vi "Actor Core.vi"(8 "error in":errorcluster, 11 "Form Model in":refnum<class "Form Model.lvclass">) -> (0 "error out":errorcluster, 3 "Actor out":refnum<class "Actor.lvclass">)   [LabVIEW 2020, in "Form Model.lvlib" / "Form Model.lvclass"]
doc: "(<B>Filename</B>: Actor Framework.lvlib:Actor.lvclass:Actor Core.vi)\n\nReceives messages to the actor, reacts to them, and initiates any error handling that may shut the actor down.\n\nDescendant classes may override this VI to append parallel tasks for the actor to complete while it handles messages. Overrides use the Call Parent Class Method node."
uses:
  Form Model.lvclass
  C:/Program Files (x86)/National Instruments/LabVIEW 2020/vi.lib/ActorFramework/Actor/Actor.lvclass
  <vilib>/ActorFramework/Actor/Actor.lvclass
  Form Model.lvclass/Form Model.ctl
  Forms Controller/Form Controller/Panel Form Controller.lvclass
  C:/Program Files (x86)/National Instruments/LabVIEW 2020/vi.lib/MGI/Panel Manager/Panel Actor/Panel Actor/Panel Actor.lvclass
  <vilib>/MGI/Panel Manager/Panel Actor/Panel Actor/Launch as Nested Actor.vi
  Form Model Configuration/Form Model Configuration Class/Form Model Configuration.lvclass
  Form Model Interfaces/Model Panel Logic Interface/Model Panel Logic.lvclass
  <vilib>/MGI/Monitored Actor/Monitored Actor/Monitored Actor/Monitored Actor.lvclass
  <vilib>/MGI/Panel Manager/Panel Actor/Panel Actor/Panel Actor.lvclass
  C:/Program Files (x86)/National Instruments/LabVIEW 2020/vi.lib/MGI/Monitored Actor/Monitored Actor/Monitored Actor/Monitored Actor.lvclass
  C:/Users/User/Desktop/Raman Program/Database OOP/source/Forms AF/Forms Controller/Form Controller/Panel Form Controller.lvclass
  C:/Users/User/Desktop/Raman Program/Database OOP/source/Forms AF/Forms Model/Form Model Actor/Form Model.lvclass
  C:/Users/User/Desktop/Raman Program/Database OOP/source/Forms AF/Forms Model/Form Model Interfaces/Form Model Messages/Form Model Messages.lvclass
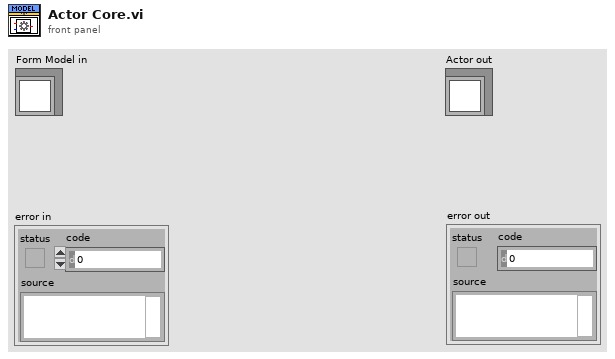
[diagram p1: front panel]
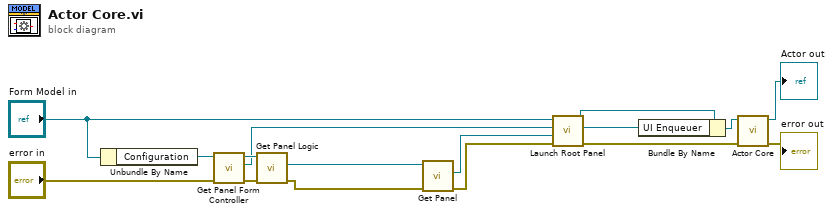
[diagram p0: block diagram]
diagram:
  n1 = Unbundle By Name("Form Model in") -> ("Configuration"=w7:refnum<class "Form Model Configuration.lvclass">)
  n2 = call-dynamic "Get Panel Form Controller.vi"("error in (no error)"="error in", "Form Model Configuration in"=w7) -> ("error out"=w5:errorcluster, "Panel Form Controller"=w8:refnum<class "Panel Form Controller.lvclass">, "Form Model Configuration out"=w9:refnum<class "Form Model Configuration.lvclass">)  [unwired: 7 in]
  n3 = call-dynamic "Get Panel Logic.vi"("error in (no error)"=w5, "Form Model Configuration in"=w9) -> ("error out"=w2:errorcluster, "Panel Logic"=w4:refnum<class "Model Panel Logic.lvclass">)  [unwired: 7 in, 1 out]
  n4 = call-dynamic "Get Panel.vi"("error in (no error)"=w2, "Model Panel Logic in"=w4) -> ("error out"=w1:errorcluster, "Panel"=w3:refnum<class "Panel.lvclass">)  [unwired: 7 in, 1 out]
  n5 = call-poly <vilib>:"Launch Root Panel.vi"("Error In"=w1, "Panel"=w3, "Panel Actor in"=w8, "Caller Actor in"="Form Model in") -> ("Error Out"=w10:errorcluster, "Actor's Enqueuer"=w12:refnum<class "Message Enqueuer.lvclass">, "Caller Actor out"=w13:refnum<class "Form Model.lvclass">)  [unwired: 5 in]
  n6 = Bundle By Name(cluster=w13, "UI Enqueuer"=w12) -> (w11:refnum<class "Form Model.lvclass">)
  n7 = call-parent "Actor Core.vi"("error in"=w10, "Actor in"=w11) -> ("error out"=→"error out":errorcluster, "Actor out"=→"Actor out":refnum<class "Actor.lvclass">)  [unwired: 8 in]
